vi "getCapacitance.vi"(8 "error in (no error)":errorcluster, 11 "Inst.AH2500 in":refnum<class "Inst.AH2500.lvclass">) -> (0 "error out":errorcluster, 2 "Capacitance (pF)":dbl, 3 "Inst.AH2500 out":refnum<class "Inst.AH2500.lvclass">)   [LabVIEW 2019, in "Inst.AH2500.lvclass"]
uses:
  Inst.AH2500.lvclass
  C:/Program Files (x86)/National Instruments/LabVIEW 2019/user.lib/LevyLab/Instrument Framework/Instrument/Instrument.lvclass
  Typedefs/Inst.AH2500.Commands--Enum.ctl
  Typedefs/Inst.AH2500.getAll--Cluster.ctl
  991804cd-2d63-4689-a149-8f7b841441b7.vi
  991804cd-2d63-4689-a149-8f7b841441b7.vi/80798ebf-8349-4e87-986d-8f50210e2eac.vi
  991804cd-2d63-4689-a149-8f7b841441b7.vi/80798ebf-8349-4e87-986d-8f50210e2eac.vi/d8c36cce-16e7-4967-9341-593f436ffed8.vi
  991804cd-2d63-4689-a149-8f7b841441b7.vi/80798ebf-8349-4e87-986d-8f50210e2eac.vi/0e276b30-0bec-4946-a8ef-b362e89b0af1.vi
  <userlib>/LevyLab/Instrument Framework/Instrument/API/Remote Client.vi
  <vilib>/Utility/Data Type/Get Type Information.vi
  <vilib>/JDP Science/JSONtext/JSON text to Variant.vi
  <vilib>/JDP Science/JSONtext/LVClass Serializer/JSONtext LVClass Serializer.lvclass
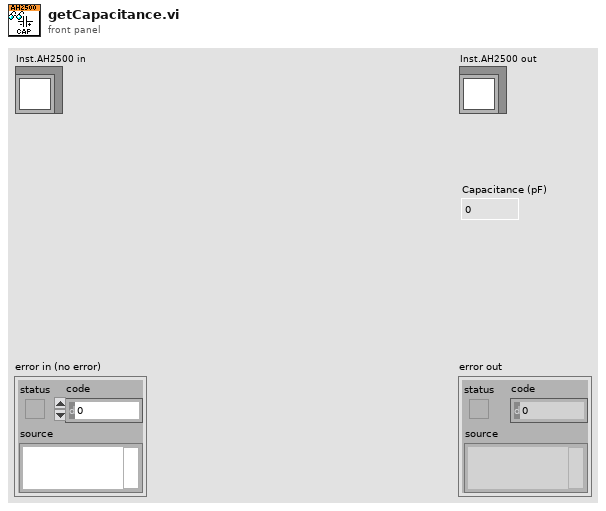
[diagram p1: front panel]
types:
  T1 = typedef "Inst.AH2500.lvclass/Inst.AH2500.getAll--Cluster.ctl" = cluster{"capacitance (pF)":dbl, "loss (nS)":dbl, "Vexc (V)":dbl}
  T2 = typedef "Inst.AH2500.lvclass/Inst.AH2500.Commands--Enum.ctl" = enum16{"getCapacitance", "getLoss", "getExcitation"}
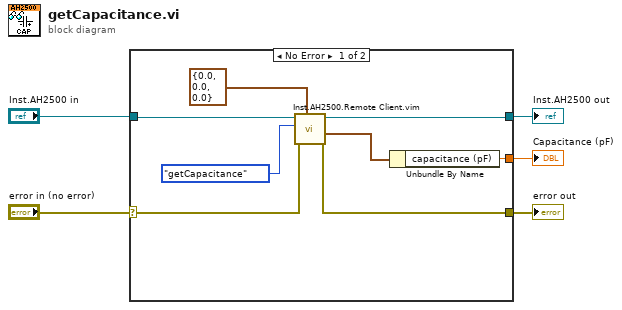
[diagram p0: block diagram]
diagram:
  n1 = case shown="No Error" "error in (no error)" {
    selector: "error in (no error)" -> [w9 w15]
    tunnel: [w6 w15] -> w4
    tunnel: [w7 w14] -> w3
    tunnel: [w13 _] -> w2
    tunnel: "Inst.AH2500 in" -> [w12 w14]
    frame No Error {
      n2 = call "Inst.AH2500.Remote Client.vim"("Data Out type"=T1 {"capacitance (pF)"=0.0, "loss (nS)"=0.0, "Vexc (V)"=0.0} ("getAll"), "error in (no error)"=w9, "Commands"=Inst.AH2500.Commands--Enum."getCapacitance", "Inst.AH2500 in"=w12) -> ("error out"=w6:errorcluster, "Data out"=w8:T1, "Inst.AH2500 out"=w7:refnum<class "Inst.AH2500.lvclass">)  [unwired: 5 in]
      n3 = Unbundle By Name(w8) -> ("capacitance (pF)"=w13:dbl)
    }
    frame Error {
    }
  }
  "error out" <- w4
  "Inst.AH2500 out" <- w3
  "Capacitance (pF)" <- w2
